vi "Interpola-V-B.vi"(7 "Modo":enum16{"Volt to Tesla", "Tesla to Volt"}(ring), 8 "error in (no error)":errorcluster, 9 "INPUT":dbl, 10 "Gap":enum16{"gap 31mm", "gap 76 mm"}(ring), 11 "FilePath":path=path "C:/Users/pemar/Documents/LabVIEW Data/XImanCalibre.txt") -> (0 "error out":errorcluster, 1 "OUTPUT":dbl)   [LabVIEW 2017]
uses:
  <vilib>/Utility/file.llb/Read Delimited Spreadsheet (string).vi
panel:
  out "V(B)gap76":string[](array[string])
  out "V(B)gap31":string[](array[string])
  out "B(V)gap76":string[](array[string])
  out "B(V)gap31":string[](array[string])
  out "AllRows":string[][](array[string])
  # "C:\\Users\\usuario\\Documents\\LabVIEW Data\\XImanCalibre.txt"
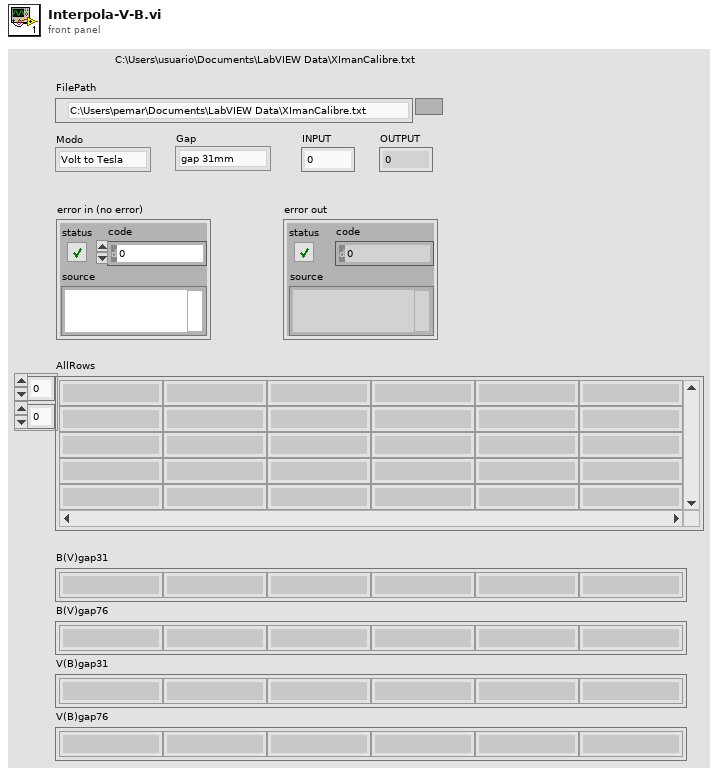
[diagram p1: front panel]
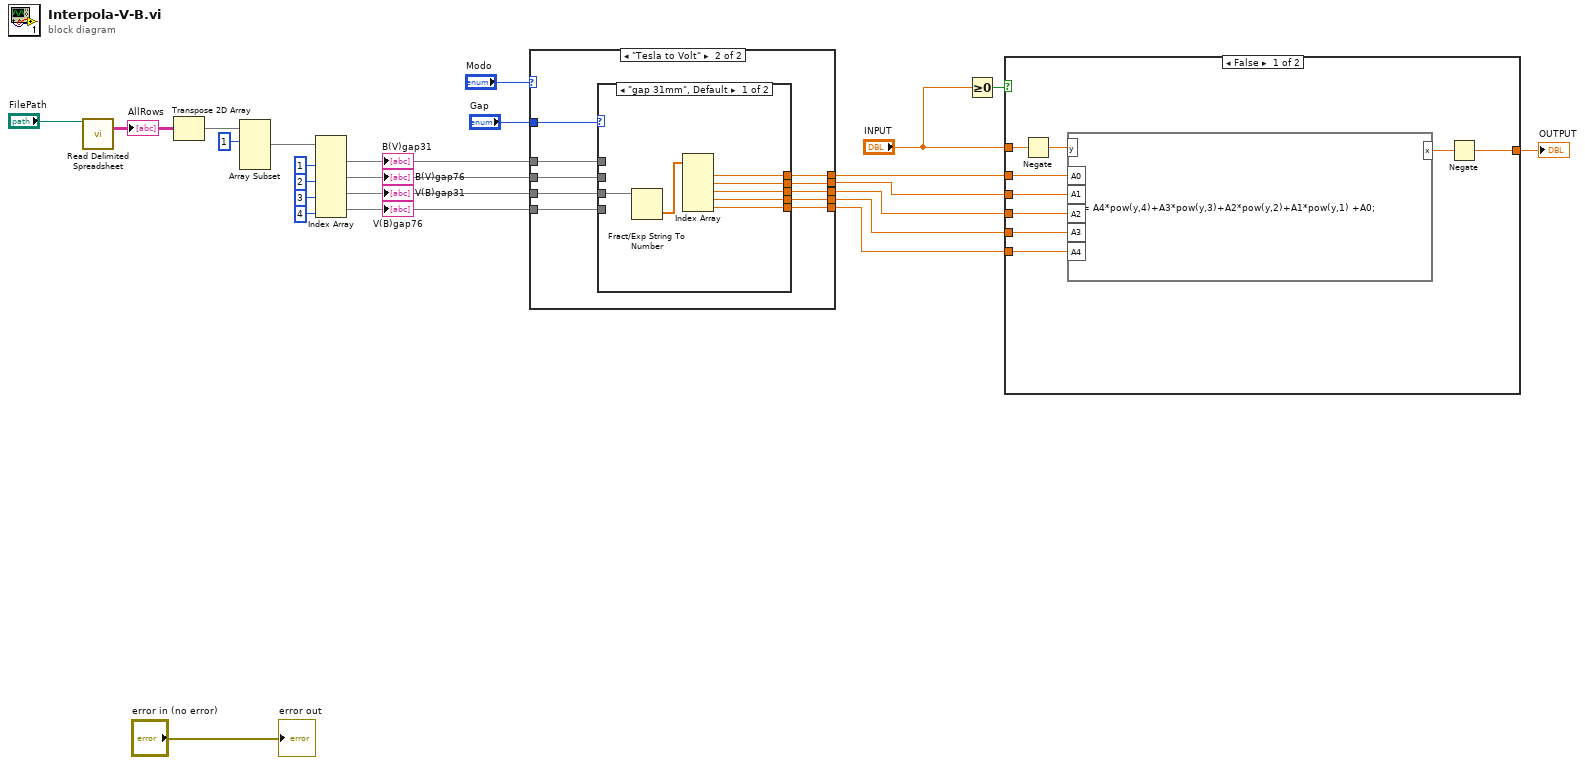
[diagram p0: block diagram]
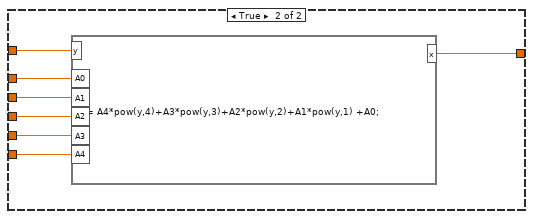
[diagram p2: hidden frame]
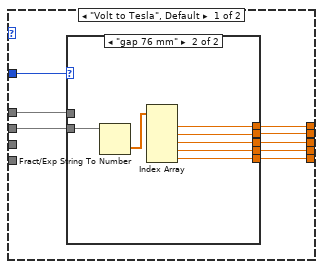
[diagram p3: hidden frame]
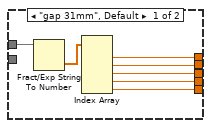
[diagram p4: hidden frame]
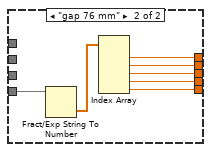
[diagram p5: hidden frame]
diagram:
  n1 = call-poly <vilib>:"Read Delimited Spreadsheet.vi"("file path (dialog if empty)"="FilePath") -> ("all rows"=w17:string[][])  [unwired: 9 in, 5 out]
  "AllRows" <- w17
  n2 = Transpose 2D Array(2D array=w17) -> (transposed array=w16:string[][])
  n3 = Array Subset(array=w16, index (row)=1 ("index")) -> (w14:string[][])  [unwired: 3 in]
  n4 = Index Array(array=w14, index (col) #1=1 ("disabled index (col)"), index (col) #2=2 ("index (col)"), index (col) #3=3 ("index (col)"), index (col) #4=4 ("index (col)")) -> (element #1=w12:string[], element #2=w11:string[], element #3=w10:string[], element #4=w9:string[])  [unwired: 4 in]
  "B(V)gap31" <- w12
  "B(V)gap76" <- w11
  "V(B)gap31" <- w10
  "V(B)gap76" <- w9
  n5 = case shown="\"Tesla to Volt\"" "Modo" {
    tunnel: w12 -> [w31 w56]
    tunnel: w11 -> [w25 w55]
    tunnel: w10 -> [_ w54]
    tunnel: w9 -> [_ w53]
    tunnel: "Gap" -> [w32 w52]
    tunnel: [w30 w51] -> w7
    tunnel: [w29 w47] -> w6
    tunnel: [w28 w48] -> w5
    tunnel: [w27 w49] -> w4
    tunnel: [w26 w50] -> w3
    frame "Volt to Tesla", Default {
      n6 = case shown="\"gap 76 mm\"" w32 {
        tunnel: w31 -> [w34 _]
        tunnel: [w39 w46] -> w30
        tunnel: [w38 w45] -> w29
        tunnel: [w37 w44] -> w28
        tunnel: [w36 w43] -> w27
        tunnel: [w35 w42] -> w26
        tunnel: w25 -> [_ w41]
        frame "gap 31mm", Default {
          n7 = Fract/Exp String To Number(string=w34) -> (number=w33:dbl[])  [unwired: 3 in, 1 out]
          n8 = Index Array(array=w33) -> (element #1=w39:dbl, element #2=w38:dbl, element #3=w37:dbl, element #4=w36:dbl, element #5=w35:dbl)  [unwired: 5 in]
        }
        frame "gap 76 mm" {
          n9 = Fract/Exp String To Number(string=w41) -> (number=w40:dbl[])  [unwired: 3 in, 1 out]
          n10 = Index Array(array=w40) -> (element #1=w46:dbl, element #2=w45:dbl, element #3=w44:dbl, element #4=w43:dbl, element #5=w42:dbl)  [unwired: 5 in]
        }
      }
    }
    frame "Tesla to Volt" {
      n11 = case shown="\"gap 31mm\", Default" w52 {
        tunnel: w56 -> [_ _]
        tunnel: w55 -> [_ _]
        tunnel: w54 -> [w58 _]
        tunnel: w53 -> [_ w65]
        tunnel: [w63 w70] -> w51
        tunnel: [w62 w69] -> w47
        tunnel: [w61 w68] -> w48
        tunnel: [w60 w67] -> w49
        tunnel: [w59 w66] -> w50
        frame "gap 31mm", Default {
          n12 = Fract/Exp String To Number(string=w58) -> (number=w57:dbl[])  [unwired: 3 in, 1 out]
          n13 = Index Array(array=w57) -> (element #1=w63:dbl, element #2=w62:dbl, element #3=w61:dbl, element #4=w60:dbl, element #5=w59:dbl)  [unwired: 5 in]
        }
        frame "gap 76 mm" {
          n14 = Fract/Exp String To Number(string=w65) -> (number=w64:dbl[])  [unwired: 3 in, 1 out]
          n15 = Index Array(array=w64) -> (element #1=w70:dbl, element #2=w69:dbl, element #3=w68:dbl, element #4=w67:dbl, element #5=w66:dbl)  [unwired: 5 in]
        }
      }
    }
  }
  n16 = Greater Or Equal To 0?(x="INPUT") -> (x >= 0?=w2:bool)
  n17 = case shown="False" w2 {
    tunnel: "INPUT" -> [w79 w86]
    tunnel: [w71 w85] -> w13
    tunnel: w7 -> [w77 w84]
    tunnel: w6 -> [w76 w83]
    tunnel: w5 -> [w75 w82]
    tunnel: w4 -> [w74 w81]
    tunnel: w3 -> [w73 w80]
    frame False {
      n18 = Negate(x=w79) -> (-x=w72:dbl)
      n19 = formula code="x= A4*pow(y,4)+A3*pow(y,3)+A2*pow(y,2)+A1*pow(y,1) +A0;"("A0"=w77, "A1"=w76, "A2"=w75, "A3"=w74, "A4"=w73, "y"=w72) -> ("x"=w78:dbl)
      n20 = Negate(x=w78) -> (-x=w71:dbl)
    }
    frame True {
      n21 = formula code="x= A4*pow(y,4)+A3*pow(y,3)+A2*pow(y,2)+A1*pow(y,1) +A0;"("A0"=w84, "A1"=w83, "A2"=w82, "A3"=w81, "A4"=w80, "y"=w86) -> ("x"=w85:dbl)
    }
  }
  "OUTPUT" <- w13
  "error out" <- "error in (no error)"
